vi "ChangeClimb.vi"(1 "Mid":bool, 2 "Low":bool) -> ()   [LabVIEW 2020]
uses:
  <vilib>/Rock Robotics/Network Tables/NT Write String.vi
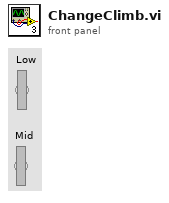
[diagram p1: front panel]
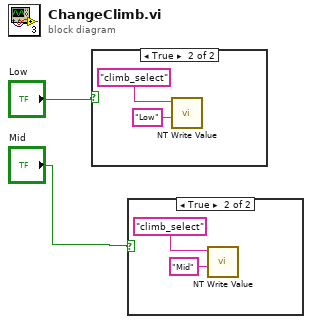
[diagram p0: block diagram]
diagram:
  n1 = case shown="True" "Low" {
    frame False {
    }
    frame True {
      n2 = call-poly <vilib>:"NT Write Value.vi"("String"="Low", "Name"="climb_select") -> ()  [unwired: 9 in, 1 out]
    }
  }
  n3 = case shown="True" "Mid" {
    frame False {
    }
    frame True {
      n4 = call-poly <vilib>:"NT Write Value.vi"("String"="Mid", "Name"="climb_select") -> ()  [unwired: 9 in, 1 out]
    }
  }
